vi "binary_reader_error_search.vi"(7 "error in":errorcluster, 10 "path to binary file":path) -> (0 "error out":errorcluster, 2 "voltage over time":waveform(dbl)(graph), 3 "3 axis acceleration in time":waveform(dbl)[](graph))   [LabVIEW 2017]
uses:
  Controls/control_time_informations.ctl
  Controls/control_measurement_settings.ctl
  Controls/control_memory_structure.ctl
  Controls/control_all_in_one_package.ctl
  Controls/control_measurement_data.ctl
panel:
  out "magnitude of acceleration vectors":waveform(dbl)(graph)
  out "Misc":T3 {"time informations"."length" format="%<%H:%M:%S%3u>t"; "actigraph settings"."id" format="%02d"; "actigraph settings"."range code" format="%02x"; "actigraph settings"."rate code" format="%02x"}
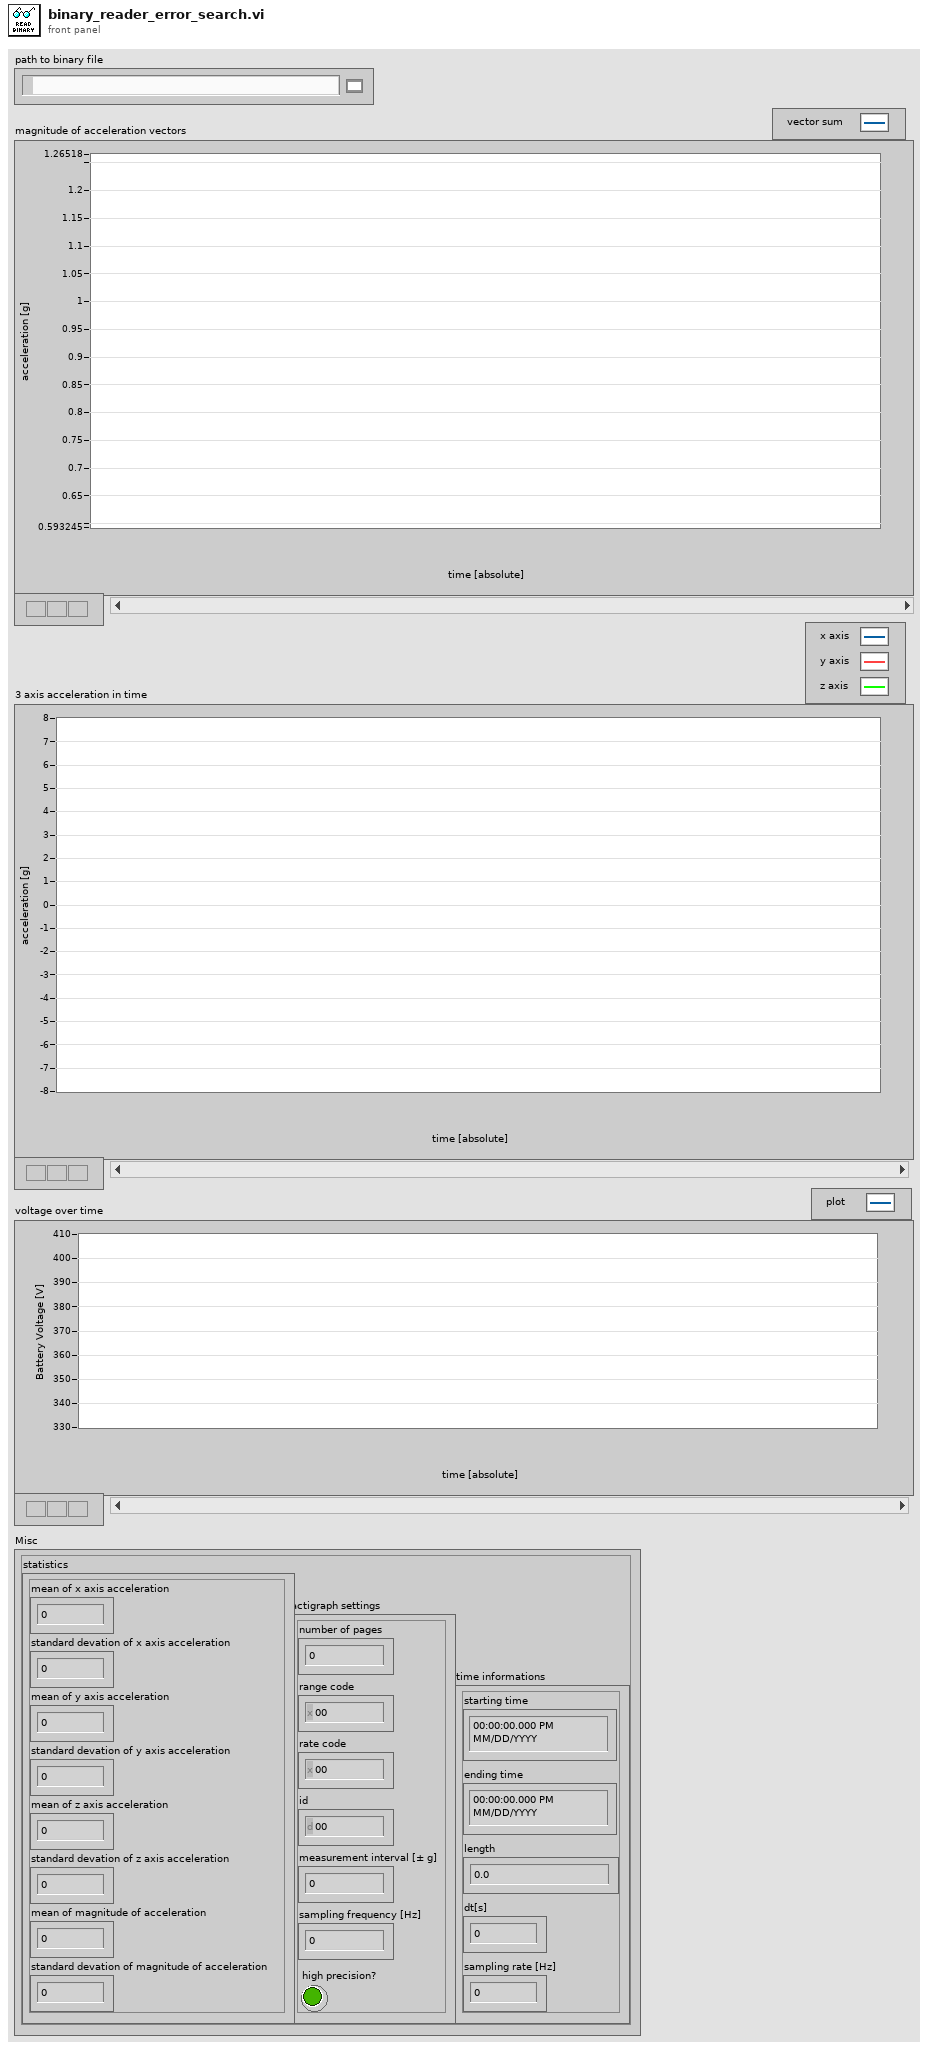
[diagram p1: front panel]
types:
  T1 = typedef "control_time_informations.ctl" = cluster{"starting time":timestamp, "ending time":timestamp, "dt[s]":dbl, "sampling rate [Hz]":dbl, "length":dbl}
  T2 = typedef "control_measurement_settings.ctl" = cluster{"sampling frequency [Hz]":dbl, "measurement interval [± g]":i32, "high precision?":bool, "number of pages":i32, "rate code":i32, "range code":i32, "id":i32}
  T3 = cluster{"statistics":cluster{"mean of x axis acceleration":dbl, "standard devation of x axis acceleration":dbl, "mean of y axis acceleration":dbl, "standard devation of y axis acceleration":dbl, "mean of z axis acceleration":dbl, "standard devation of z axis acceleration":dbl, "mean of magnitude of acceleration":dbl, "standard devation of magnitude of acceleration":dbl}, "time informations":T1, "actigraph settings":T2}
  T4 = typedef "control_memory_structure.ctl" = cluster{"length of metadata [byte]":i32, "length of page [byte]":i32, "length of measurement \ndata on page [byte]":i32, "length of dataset [byte]":i32}
  T5 = typedef "control_all_in_one_package.ctl" = cluster{"measurement data":T6, "actigraph settings":T2, "memory structure":T4, "time informations":T1}
  T6 = typedef "control_measurement_data.ctl" = cluster{"number of samples per axis":i32, "timestamp array":dbl[], "offset array":dbl[], "x, y, z axis data":waveform(dbl)[], "magnitude of acceleartion vectors":waveform(dbl), "statistics":cluster{"mean of x axis acceleration":dbl, "standard devation \nof x axis acceleration":dbl, "mean of y axis acceleration":dbl, "standard devation \nof y axis acceleration":dbl, "mean of z axis acceleration":dbl, "standard devation \nof z axis acceleration":dbl, "mean of magnitude\n of acceleration":dbl, "standard devation \nof magnitude of acceleration":dbl}, "voltage":waveform(dbl)}
  T7 = cluster{"mean of x axis acceleration":dbl, "standard devation \nof x axis acceleration":dbl, "mean of y axis acceleration":dbl, "standard devation \nof y axis acceleration":dbl, "mean of z axis acceleration":dbl, "standard devation \nof z axis acceleration":dbl, "mean of magnitude\n of acceleration":dbl, "standard devation \nof magnitude of acceleration":dbl}
  T8 = cluster{"mean of x axis acceleration":dbl, "standard devation of x axis acceleration":dbl, "mean of y axis acceleration":dbl, "standard devation of y axis acceleration":dbl, "mean of z axis acceleration":dbl, "standard devation of z axis acceleration":dbl, "mean of magnitude of acceleration":dbl, "standard devation of magnitude of acceleration":dbl}
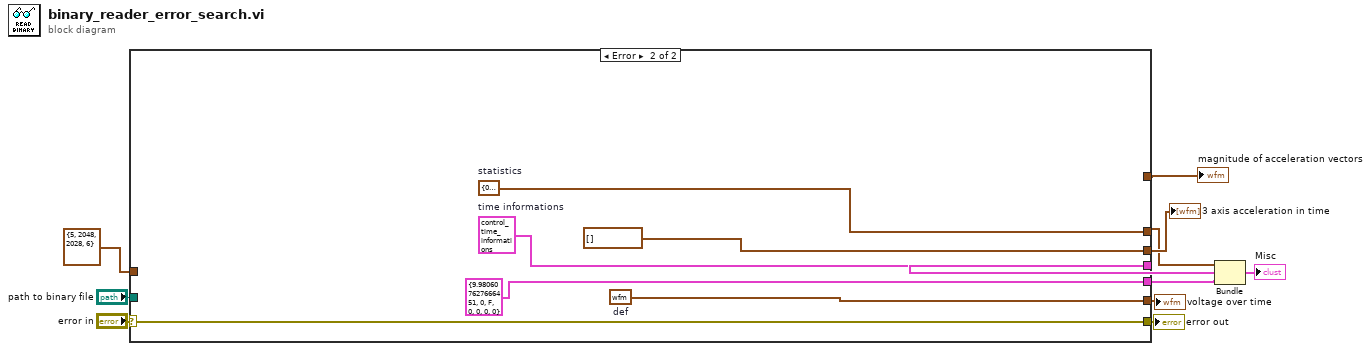
[diagram p0: block diagram]
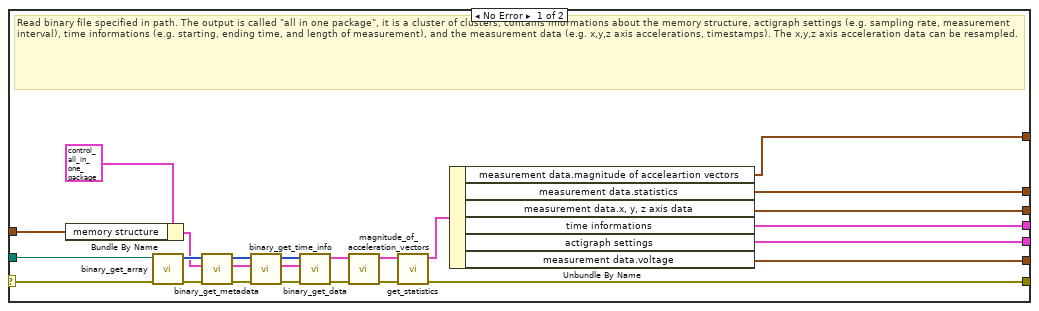
[diagram p2: hidden frame]
diagram:
  n1 = case shown="Error" "error in" {
    selector: "error in" -> [w22 w42]
    tunnel: "path to binary file" -> [w35 _]
    tunnel: T4 {"length of metadata [byte]"=5, "length of page [byte]"=2048, "length of measurement \ndata on page [byte]"=2028, "length of dataset [byte]"=6} ("memory structure") -> [w29 _]
    tunnel: [w17 w42] -> w10
    tunnel: [w28 waveform(dbl)[] [] ("x, y, z axis data")] -> w7
    tunnel: [w25 w40] -> w4
    tunnel: [w24 T2 {"sampling frequency [Hz]"=9.980607627666451, "measurement interval [± g]"=0, "high precision?"=FALSE, "number of pages"=0, "rate code"=0, "range code"=0, "id"=0} ("actigraph settings")] -> w3
    tunnel: [w18 w38] -> w5
    tunnel: [w13 w37] -> w6
    tunnel: [w12 _] -> w1
    frame No Error {
      # "Read binary file specified in path. The output is called \"all in one package\", it is a cluster of clusters, contains informations about the memory structure, actigraph settings (e.g. sampling rate, measurement interval), time informations (e.g. starting, ending time, and length of measurement), and the measurement data (e.g. x,y,z axis accelerations, timestamps). The x,y,z axis acceleration data can be resampled."
      n2 = Bundle By Name(cluster=T5 {"measurement data"={"number of samples per axis"=0, "timestamp array"=[], "offset array"=[], "x, y, z axis data"=[], "magnitude of acceleartion vectors"={"t0"=timestamp(0 s since 1904-01-01), "dt"=1.0, "Y"=[]}, "statistics"={"mean of x axis acceleration"=0.0, "standard devation \nof x axis acceleration"=0.0, "mean of y axis acceleration"=0.0, "standard devation \nof y axis acceleration"=0.0, "mean of z axis acceleration"=0.0, "standard devation \nof z axis acceleration"=0.0, "mean of magnitude\n of acceleration"=0.0, "standard devation \nof magnitude of acceleration"=0.0}, "voltage"={"t0"=timestamp(0 s since 1904-01-01), "dt"=1.0, "Y"=[]}}, "actigraph settings"={"sampling frequency [Hz]"=0.0, "measurement interval [± g]"=0, "high precision?"=FALSE, "number of pages"=0, "rate code"=0, "range code"=0, "id"=0}, "memory structure"={"length of metadata [byte]"=0, "length of page [byte]"=0, "length of measurement \ndata on page [byte]"=0, "length of dataset [byte]"=0}, "time informations"={"starting time"=timestamp(0 s since 1904-01-01), "ending time"=timestamp(0 s since 1904-01-01), "dt[s]"=0.0, "sampling rate [Hz]"=0.0, "length"=0.0}} ("all in one package"), "memory structure"=w29) -> (w26:T5)
      n3 = call "binary_get_array.vi"("error in"=w22, "path to binary file"=w35) -> ("error out"=w34:errorcluster, "binary data"=w32:u8[])  [unwired: 8 in]
      n4 = call "binary_get_metadata.vi"("error in"=w34, "all in one package in"=w26, "binary data"=w32) -> ("error out"=w36:errorcluster, "all in one package out"=w27:T5, "pages"=w33:u8[])  [unwired: 6 in]
      n5 = call "binary_get_time_info.vi"("error in"=w36, "all in one package in"=w27, "pages"=w33) -> ("error out"=w31:errorcluster, "all in one package out"=w23:T5, "pages excluding first and last page"=w30:u8[])  [unwired: 6 in]
      n6 = call "binary_get_data.vi"("error in"=w31, "all in one package in"=w23, "pages excluding first and last page"=w30) -> ("error out"=w21:errorcluster, "all in one package out"=w16:T5)  [unwired: 7 in]
      n7 = call "magnitude_of_acceleration_vectors.vi"("error in"=w21, "all in one package in"=w16) -> ("error out"=w20:errorcluster, "all in one package out"=w19:T5)  [unwired: 8 in]
      n8 = call "get_statistics.vi"("error in"=w20, "all in one package in"=w19) -> ("error out"=w17:errorcluster, "all in one package out"=w15:T5)  [unwired: 8 in]
      n9 = Unbundle By Name(w15) -> ("measurement data.magnitude of acceleartion vectors"=w12:waveform(dbl), "measurement data.statistics"=w18:T7, "measurement data.x, y, z axis data"=w28:waveform(dbl)[], "time informations"=w25:T1, "actigraph settings"=w24:T2, "measurement data.voltage"=w13:waveform(dbl))
    }
    frame Error {
      w37 = waveform(dbl) {"t0"=timestamp(0 s since 1904-01-01), "dt"=1.0, "Y"=[]}  # def
      w38 = T8 {"mean of x axis acceleration"=0.0, "standard devation of x axis acceleration"=0.0, "mean of y axis acceleration"=0.0, "standard devation of y axis acceleration"=0.0, "mean of z axis acceleration"=0.0, "standard devation of z axis acceleration"=0.0, "mean of magnitude of acceleration"=0.0, "standard devation of magnitude of acceleration"=0.0}  # statistics
      w40 = T1 {"starting time"=timestamp(0 s since 1904-01-01), "ending time"=timestamp(0 s since 1904-01-01), "dt[s]"=0.0, "sampling rate [Hz]"=0.0, "length"=0.0}  # time informations
    }
  }
  "error out" <- w10
  "3 axis acceleration in time" <- w7
  "voltage over time" <- w6
  "magnitude of acceleration vectors" <- w1
  n10 = Bundle("statistics"=w5, "time informations"=w4, "actigraph settings"=w3) -> (→"Misc":T3)  [unwired: 1 in]
